vi "Retract.vi"(8 "Reset":bool, 9 "Shooter Sensor":bool, 10 "Arm Up Sensor":bool) -> (0 "Shooter Motor":dbl, 1 "Finished":bool, 3 "Arm":T1)   [LabVIEW 2013]
uses:
  <vilib>/Rock Robotics/WPI/Solenoid/WPI_SolenoidValue.ctl
  Retract States.ctl
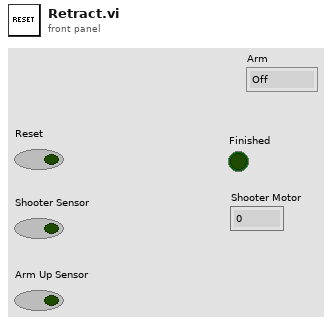
[diagram p1: front panel]
types:
  T1 = typedef "WPI_SolenoidValue.ctl" = enum16{"Off", "On", "Forward", "Reverse"}
  T2 = typedef "Retract States.ctl" = enum16{"Arm Shooter", "Retract Arm", "Finished"}
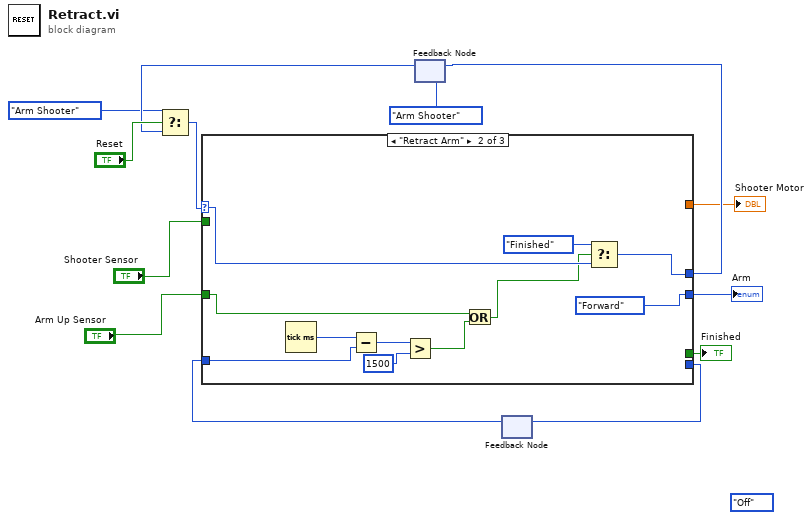
[diagram p0: block diagram]
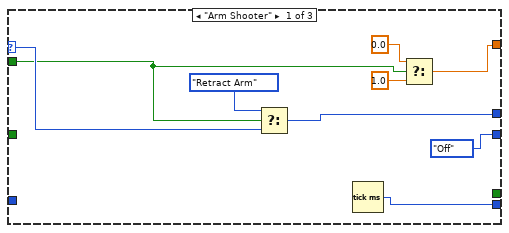
[diagram p2: hidden frame]
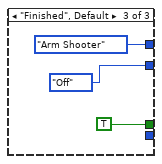
[diagram p3: hidden frame]
diagram:
  (unwired) WPI_SolenoidValue."Off" ("Arm State")
  n1 = feedback #1(Retract_States."Arm Shooter" ("Enum")) -> (w6:T2)
  n2 = Select(t=Retract_States."Arm Shooter" ("Enum"), s="Reset", f=w6) -> (s? t:f=w4:T2)
  n3 = feedback #2() -> (w1:u32)  [unwired: 1 in]
  n4 = case shown="\"Retract Arm\"" w4 {
    selector: w4 -> [w22 w32 _]
    tunnel: [w21 w33 Retract_States."Arm Shooter" ("Enum")] -> w12
    tunnel: [WPI_SolenoidValue."Off" ("Arm State") WPI_SolenoidValue."Forward" ("Arm State") WPI_SolenoidValue."Off" ("Arm State")] -> w11
    tunnel: "Shooter Sensor" -> [w15 _ _]
    tunnel: "Arm Up Sensor" -> [_ w25 _]
    tunnel: [_ _ TRUE ("Finished")] -> w8
    tunnel: [w16 _ _] -> w3
    tunnel: [w14 _ _] -> w2
    tunnel: w1 -> [_ w28 _]
    frame "Arm Shooter" {
      n5 = Select(t=Retract_States."Retract Arm", s=w15, f=w22) -> (s? t:f=w21:T2)
      n6 = Tick Count (ms)() -> (millisecond timer value=w14:u32)
      n7 = Select(t=0.0, s=w15, f=1.0) -> (s? t:f=w16:dbl)
    }
    frame "Retract Arm" {
      n8 = Tick Count (ms)() -> (millisecond timer value=w29:u32)
      n9 = Subtract(x=w29, y=w28) -> (x-y=w27:u32)
      n10 = Greater?(x=w27, y=u32 1500) -> (0:w24:bool)
      n11 = Or(x=w25, y=w24) -> (x .or. y?=w23:bool)
      n12 = Select(t=Retract_States."Finished", s=w23, f=w32) -> (s? t:f=w33:T2)
    }
    frame "Finished", Default {
    }
  }
  "Shooter Motor" <- w3
  "Finished" <- w8
  "Arm" <- w11
  n13 = feedback-in #1(w12) -> ()
  n14 = feedback-in #2(w2) -> ()
